vi "JSON Schema to Table.vi"(8 "error in (no error)":errorcluster, 11 "JSON Schema in":string) -> (0 "error out":errorcluster, 2 "Table":string[][](table), 3 "JSON Schema out":string)   [LabVIEW 2019, in "JSON-Schema.lvlib"]
uses:
  JSON-Schema.lvlib
  a58aa99b-14ca-48af-b081-8c0a9da57a3d.vi
  fd2d87a8-6ab4-473d-a4e8-527c74bc07ef.vi
  <vilib>/JDP Science/JSONtext/Next JSON Value.vi
  <vilib>/JDP Science/JSONtext/String Subset.vi
  <vilib>/JDP Science/JSONtext/Parsing/Advance past next JSON Value (inlined COPY).vi
  <vilib>/JDP Science/JSONtext/Parsing/Advance past whitespace.vi
  <vilib>/JDP Science/JSONtext/Parsing/Advance past String.vi
  <vilib>/JDP Science/JSONtext/Parsing/Advance past Number.vi
  <vilib>/JDP Science/JSONtext/Parsing/Advance past Line Ending.vi
  <vilib>/JDP Science/JSONtext/Parsing/Parse Full Path or Item Name.vi
  <vilib>/JDP Science/JSONtext/Parsing/Advance past Array.vi
  <vilib>/JDP Science/JSONtext/Parsing/Advance past Object.vi
  <vilib>/JDP Science/JSONtext/support/Error Cluster From Code.vi
  <vilib>/JDP Science/JSONtext/Offset/Find Item Locations by Path.vi
  <vilib>/JDP Science/JSONtext/JSON text to Variant.vi
  <vilib>/JDP Science/JSONtext/LVClass Serializer/JSONtext LVClass Serializer.lvclass
  <vilib>/JDP Science/JSONtext/JSONtext.lvlib
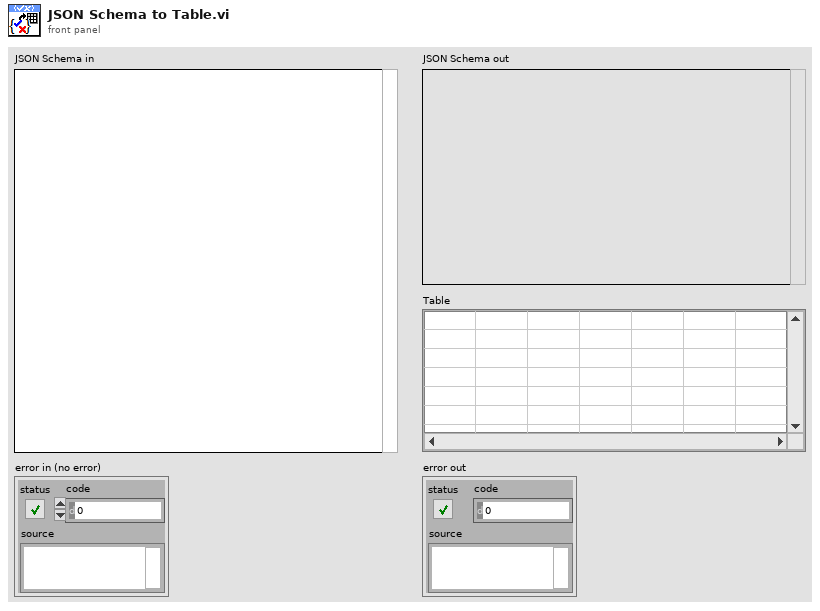
[diagram p1: front panel]
types:
  T1 = typedef "JSONtext.lvlib/JSON Value Type.ctl" = enum16{"Not a JSON Value", "JSON Object", "JSON Array", "String", "Number", "true", "false", "null"}
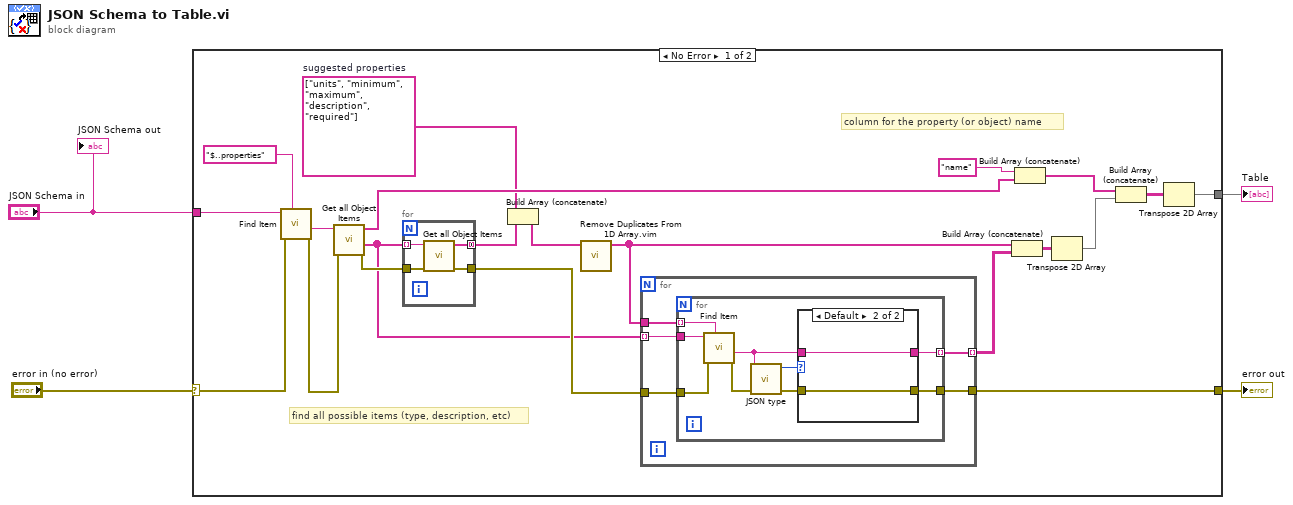
[diagram p0: block diagram]
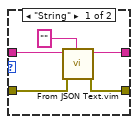
[diagram p2: hidden frame]
diagram:
  n1 = case shown="No Error" "error in (no error)" {
    selector: "error in (no error)" -> [w25 w50]
    tunnel: "JSON Schema in" -> [w24 _]
    tunnel: [w17 _] -> w3
    tunnel: [w13 w50] -> w2
    frame No Error {
      w5 = string[] ["units", "minimum", "maximum", "description", "required"]  # suggested properties
      # "column for the property (or object) name"
      # "find all possible items (type, description, etc)"
      n2 = call <vilib>:"Find Item.vi"("$Path or Item Name"="$..properties", "error in (no error)"=w25, "JSON"=w24) -> ("error out"=w16:errorcluster, "<JSON>"=w19:string)  [unwired: 5 in, 2 out]
      n3 = call <vilib>:"Get all Object Items.vi"("error in (no error)"=w16, "JSON"=w19) -> ("error out"=w11:errorcluster, "<JSON>"=w8:string[], "Item Names"=w9:string[])  [unwired: 6 in, 1 out]
      n4 = for {
        tunnel: w8 -> [w49] mode=indexing
        tunnel: [w48] -> w7 mode=concatenating
        tunnel: w11 -> [w47]
        tunnel: [w46] -> w15
        n5 = call <vilib>:"Get all Object Items.vi"("error in (no error)"=w47, "JSON"=w49) -> ("error out"=w46:errorcluster, "Item Names"=w48:string[])  [unwired: 6 in, 2 out]
      }
      n6 = Build Array (concatenate)(w5, w7) -> (w6:string[])
      n7 = call "Remove Duplicates From 1D Array.vim"("array"=w6) -> ("array with duplicates removed"=w12:string[])  [unwired: 10 in]
      n8 = for {
        tunnel: w8 -> [w30] mode=indexing
        tunnel: w12 -> [w29]
        tunnel: [w28] -> w20 mode=indexing
        tunnel: w15 -> [w27]
        tunnel: [w26] -> w13
        n9 = for {
          tunnel: w30 -> [w38]
          tunnel: w29 -> [w34] mode=indexing
          tunnel: [w36] -> w28 mode=indexing
          tunnel: w27 -> [w32]
          tunnel: [w31] -> w26
          n10 = call <vilib>:"Find Item.vi"("$Path or Item Name"=w34, "error in (no error)"=w32, "JSON"=w38) -> ("error out"=w33:errorcluster, "<JSON>"=w35:string)  [unwired: 5 in, 2 out]
          n11 = call <vilib>:"JSON type.vi"("JSON"=w35) -> ("JSON Value Type"=w37:T1)  [unwired: 9 in, 1 out]
          n12 = case shown="Default" w37 {
            tunnel: [w43 w45] -> w36
            tunnel: w35 -> [w41 w45]
            tunnel: w33 -> [w40 w44]
            tunnel: [w39 w44] -> w31
            frame "String" {
              n13 = call "From JSON Text.vim"("Data Type and Default Value"="", "error in (no error)"=w40, "JSON"=w41) -> ("error out"=w39:errorcluster, "Data out"=w43:string)  [unwired: 7 in]
            }
            frame Default {
            }
          }
        }
      }
      n14 = Build Array (concatenate)(w12, w20) -> (w21:string[][])
      n15 = Build Array (concatenate)("name" ("$Path or Item Name"), w9) -> (w10:string[])
      n16 = Transpose 2D Array(2D array=w21) -> (transposed array=w14:string[][])
      n17 = Build Array (concatenate)(w10, w14) -> (w22:string[][])
      n18 = Transpose 2D Array(2D array=w22) -> (transposed array=w17:string[][])
    }
    frame Error {
    }
  }
  "Table" <- w3
  "error out" <- w2
  "JSON Schema out" <- "JSON Schema in"
